vi "test_ccd_chipSize.vi"(8 "error in":errorcluster, 11 "CCD in":refnum<class "CCD.lvclass">) -> (0 "error out":errorcluster, 3 "CCD out":refnum<class "CCD.lvclass">)   [LabVIEW 2023, in "horiba.test.lvlib"]
uses:
  Classes/CCD/CCD.lvclass
  horiba.test.lvlib
  <vilib>/addons/_JKI Toolkits/Caraya/classes/Test/Test.lvclass
  <vilib>/addons/_JKI Toolkits/Caraya/classes/Assert/Assert.lvclass
  <userlib>/_OpenG.lib/lvdata/lvdata.llb/openg_variant.lvlib
  C:/Projects/Horiba/horiba-labview-sdk/Source/Classes/GenericDevice/GenericDevice.lvclass
  C:/Projects/Horiba/horiba-labview-sdk/Source/Classes/CCD/CCD.lvclass
  <vilib>/addons/_JKI Toolkits/Caraya/classes/Assert/Assert Equal Value and Type_Variant.vi
panel:
  # "Connector Pane"
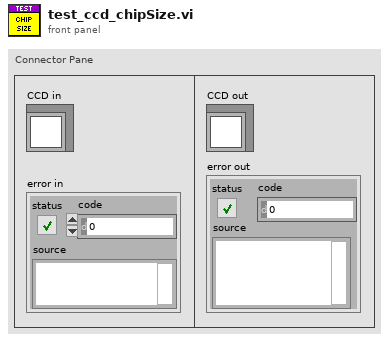
[diagram p1: front panel]
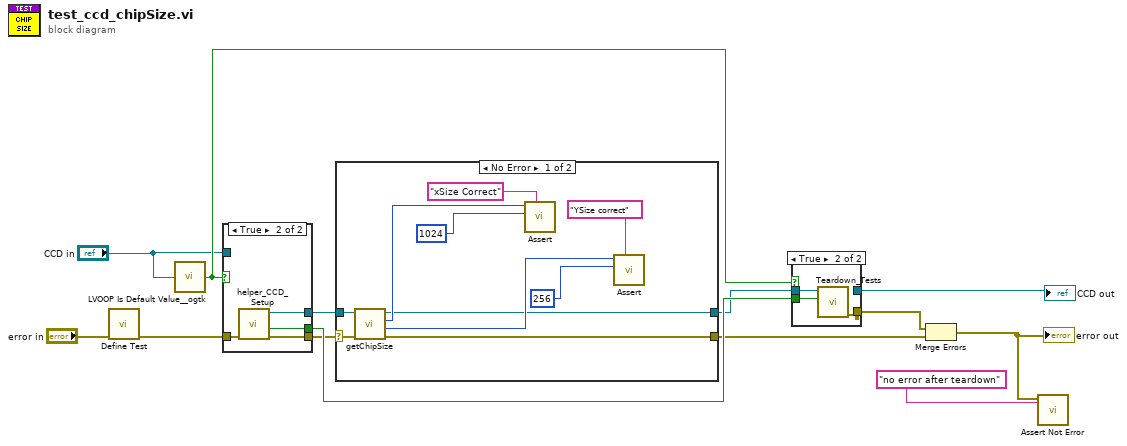
[diagram p0: block diagram]
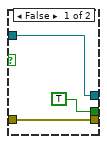
[diagram p2: hidden frame]
diagram:
  n1 = call <vilib>:"Define Test.vi"("error in (no error)"="error in") -> ("error out"=w8:errorcluster)  [unwired: 9 in, 1 out]
  n2 = call <userlib>:"LVOOP Is Default Value__ogtk.vi"("Object"="CCD in") -> ("Is Default Value?"=w9:bool)
  n3 = case shown="True" w9 {
    tunnel: w8 -> [w15 w20]
    tunnel: [w15 w19] -> w4
    tunnel: [w16 w18] -> w6
    tunnel: [TRUE ("Module Was Already Running?") w17] -> w10
    tunnel: "CCD in" -> [w16 _]
    frame False {
    }
    frame True {
      n4 = call "helper_CCD_Setup.vi"("error in"=w20) -> ("error out"=w19:errorcluster, "Module Was Already Running?"=w17:bool, "CCD out"=w18:refnum<class "CCD.lvclass">)  [unwired: 7 in, 1 out]
    }
  }
  n5 = case shown="No Error" w4 {
    selector: w4 -> [w24 w32]
    tunnel: [w22 w31] -> w5
    tunnel: w6 -> [w21 w31]
    tunnel: [w23 w32] -> w3
    frame No Error {
      n6 = call-dynamic "getChipSize.vi"("error in (no error)"=w24, "CCD in"=w21) -> ("error out"=w23:errorcluster, "chip size, y"=w30:i32, "chip size, x"=w29:i32, "CCD out"=w22:refnum<class "CCD.lvclass">)  [unwired: 6 in]
      n7 = call-poly <vilib>:"Assert.vi"("Label"="xSize Correct" ("Label (VI Title)"), "Y"=1024, "X"=w29) -> ()  [unwired: 7 in, 2 out]
      n8 = call-poly <vilib>:"Assert.vi"("Label"="YSize correct" ("Label (VI Title)"), "Y"=256, "X"=w30) -> ()  [unwired: 7 in, 2 out]
    }
    frame Error {
    }
  }
  n9 = case shown="True" w9 {
    tunnel: w5 -> [w33 w36]
    tunnel: [_ w35] -> w7
    tunnel: w10 -> [_ w34]
    tunnel: [w33 _] -> w1
    frame False {
    }
    frame True {
      n10 = call "Teardown_Tests.vi"("Module Was Already Running?"=w34, "horiba.lvlib:GenericDevice"=w36) -> ("error out"=w35:errorcluster)  [unwired: 8 in, 1 out]
    }
  }
  "CCD out" <- w1
  n11 = Merge Errors(w7, w3) -> (w12:errorcluster)
  "error out" <- w12
  n12 = call <vilib>:"Assert Not Error.vi"("Label"="no error after teardown", "Not Error?"=w12) -> ()  [unwired: 8 in, 2 out]
